vi "Place Piece.vi"(8 "error in (no error)":errorcluster caption="entrée d'erreur (pas d'erreur)", 11 "Game Board en entrée":refnum<class "Game Board.lvclass">) -> (0 "error out":errorcluster caption="sortie d'erreur", 2 "Board Full":bool, 3 "Game Board en sortie":refnum<class "Game Board.lvclass">)   [LabVIEW 2017, in "Game Board.lvclass"]
uses:
  Game Board.lvclass
  Game Board.lvclass/Game Board.ctl
  Wall_class/Wall.lvclass
  Piece of Bricks_class/Piece of Bricks.lvclass
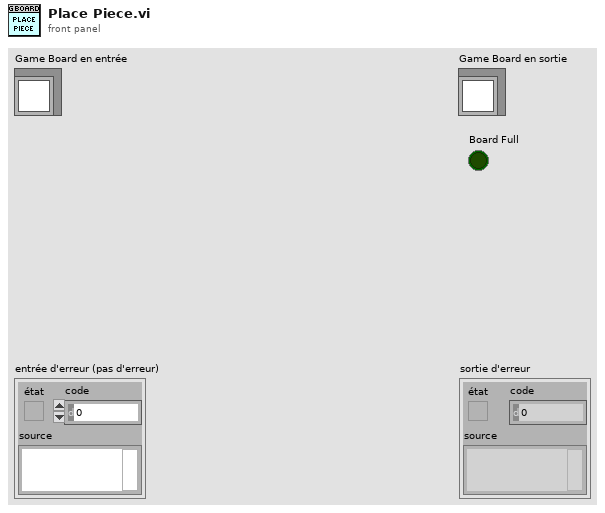
[diagram p1: front panel]
types:
  T1 = typedef "Coordinates.ctl" = cluster{"X":i32, "Y":i32}
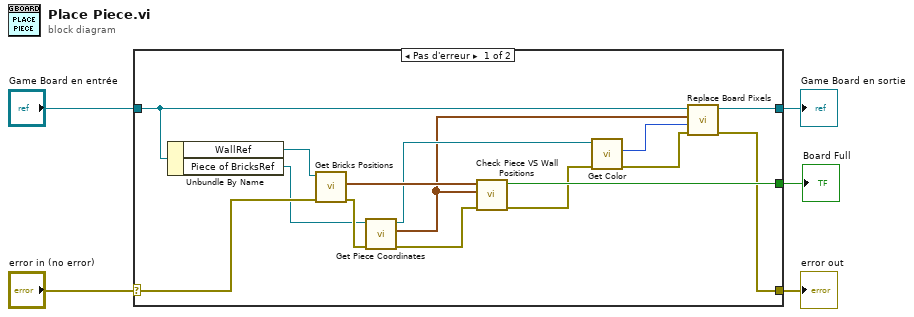
[diagram p0: block diagram]
diagram:
  n1 = case shown="Pas d'erreur" "error in (no error)" {
    selector: "error in (no error)" -> [w16 w22]
    tunnel: [w11 w22] -> w4
    tunnel: [w12 w21] -> w2
    tunnel: "Game Board en entrée" -> [w13 w21]
    tunnel: [w14 _] -> w1
    frame No Error {
      n2 = Unbundle By Name(w13) -> ("WallRef"=w18:refnum<class "Wall.lvclass">, "Piece of BricksRef"=w15:refnum<class "Piece of Bricks.lvclass">)
      n3 = call-dynamic "Get Bricks Positions.vi"("error in (no error)"=w16, "object in"=w18) -> ("error out"=w17:errorcluster, "Brick Wall"=w19:T1[])  [unwired: 7 in, 1 out]
      n4 = call-dynamic "Get Piece Coordinates.vi"("error in (no error)"=w17, "object in"=w15) -> ("error out"=w7:errorcluster, "Piece Coordinates"=w8:T1[], "object out"=w9:refnum<class "Piece of Bricks.lvclass">)  [unwired: 7 in]
      n5 = call "Check Piece VS Wall Positions.vi"("Error In"=w7, "Piece Coordinates"=w8, "Brick Wall"=w19) -> ("Error Out"=w6:errorcluster, "Invalid Move"=w14:bool)  [unwired: 7 in]
      n6 = call-dynamic "Get Color.vi"("error in (no error)"=w6, "object in"=w9) -> ("error out"=w20:errorcluster, "Color"=w10:u32)  [unwired: 7 in, 1 out]
      n7 = call-dynamic "Replace Board Pixels.vi"("error in (no error)"=w20, "New pixels color"=w10, "Pixels"=w8, "Game Board en entrée"=w13) -> ("error out"=w11:errorcluster, "Game Board en sortie"=w12:refnum<class "Game Board.lvclass">)  [unwired: 6 in]
    }
    frame Error {
    }
  }
  "error out" <- w4
  "Game Board en sortie" <- w2
  "Board Full" <- w1
